vi "Initialize Default.vi"(8 "error in (no error)":errorcluster, 11 "UDPlog Transfer Tx Configuration in":refnum<class "UDPlog Transfer Tx Configuration.lvclass">) -> (0 "error out":errorcluster, 3 "UDPlog Transfer Tx Configuration out":refnum<class "UDPlog Transfer Tx Configuration.lvclass">)   [LabVIEW 2023, in "UDPlog.lvlib" / "UDPlog Transfer Tx Configuration.lvclass"]
uses:
  UDPlog Transfer Tx Configuration.lvclass
  UDPlog Transfer Tx Configuration.lvclass/UDPlog Transfer Tx Configuration.ctl
  <vilib>/AddOns/VeriStand Custom Device Scripting APIs/Data Sharing Framework/DSF Core.lvlibp/Classes/Configuration/Configuration.lvclass
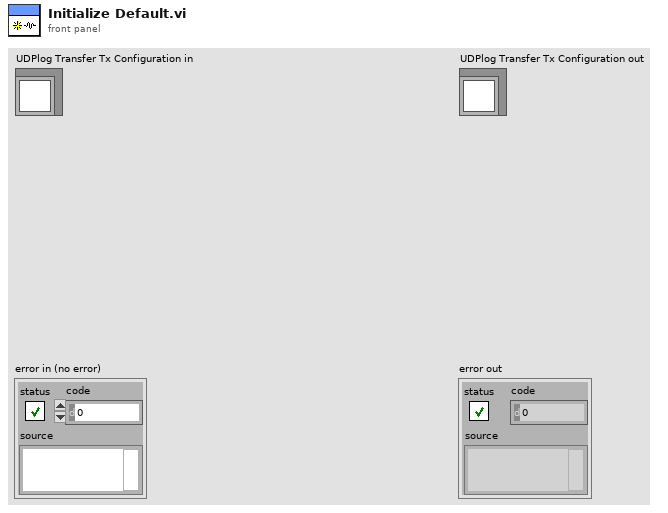
[diagram p1: front panel]
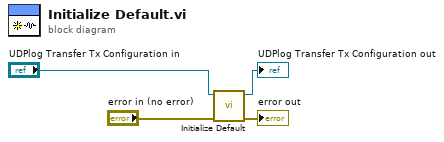
[diagram p0: block diagram]
diagram:
  n1 = call-parent "Initialize Default.vi"("error in (no error)"="error in (no error)", "Configuration in"="UDPlog Transfer Tx Configuration in") -> ("error out"=→"error out":errorcluster, "Configuration out"=→"UDPlog Transfer Tx Configuration out":refnum<class "UDPlog Transfer Tx Configuration.lvclass">)  [unwired: 8 in]
